vi "Alarm Test.vi"() -> ()   [LabVIEW 2020]
panel:
  in  "Numeric":dbl
  out "String":string
  in  "stop":bool
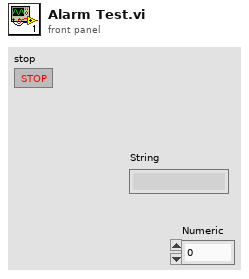
[diagram p1: front panel]
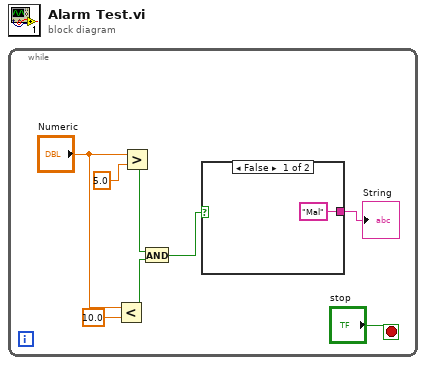
[diagram p0: block diagram]
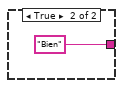
[diagram p2: hidden frame]
diagram:
  n1 = while {
    stop <- "stop" stop-if-true
    n2 = Less?(x="Numeric", y=10.0) -> (x < y?=w4:bool)
    n3 = Greater?(x="Numeric", y=5.0) -> (0:w5:bool)
    n4 = And(x=w5, y=w4) -> (x .and. y?=w6:bool)
    n5 = case shown="False" w6 {
      tunnel: ["Mal" "Bien"] -> w7
      frame False {
      }
      frame True {
      }
    }
    "String" <- w7
  }
